vi "fill the pulse memory 4 memorys.vi"(10 "memory units":T1={"Memory In"="pulse on memory", "Memory In 2"="", "Memory In 3"="", "Memory In 6"="pulse on memory"}, 11 "FIFO In":refnum<k21>="fifo pulse from host") -> ()   [LabVIEW 2021]
uses:
  <vilib>/rvi/DataTransferAndStorage/Container/Common/niFpgaContainerExecOnDevCompGetState.vi
  <vilib>/rvi/Emulation/niFpgaEmulationIsFPGAContextNoSignature.vi
  <vilib>/rvi/Emulation/niFpgaSctlEmulationGetInTimedLoop.vi
  <vilib>/rvi/errors/niFpgaSetErrorForExecOnDevCompSimple.vi
  <vilib>/rvi/eio/common/nirviEmuReportErrorAndStop.vi
  <vilib>/rvi/DataTransferAndStorage/Container/Common/niFpgaContainerGetUniqueNameForEmu.vi
  <vilib>/rvi/FIFO/Fifo_Resource/nirvififoEmulationSetSize.vi
  <vilib>/rvi/FIFO/Fifo_Resource/nirviFifoEmulationQueueMgr.vi
  <instcachedir>/0/nirviFifoEmulationQueueMgr_E5CAEC123FF24DC58D834DCA3CDAA9B5.lvgen/nirviFifoEmulationQueueMgr_E5CAEC123FF24DC58D834DCA3CDAA9B5_008.vi
  <vilib>/rvi/FIFO/Fifo_Resource/nirvififoEmulationDetermineInputValidOut.vi
  <vilib>/rvi/FIFO/Fifo_Resource/nirvififoEmulationCreateLock.vi
  <vilib>/rvi/Emulation/niFpgaProcessEmulError.vi
  <vilib>/rvi/FIFO/Fifo_Resource/nirvififoEmulationObtainLock.vi
  <vilib>/rvi/FIFO/Fifo_Resource/nirvififoEmulationReleaseLock.vi
  <vilib>/rvi/occurrence/nirviWaitOnOccurrenceBase.vi
  <vilib>/rvi/errors/nirviReportUnexpectedCaseInternalError.vi
  <vilib>/rvi/errors/nirviReportUnexpectedCaseInternalError (U32).vi
  <vilib>/Utility/error.llb/Clear Errors.vi
  <vilib>/rvi/interface/RandomDataEmulation/niFpgaRandomDataHandleErrors.vi
  <vilib>/rvi/Memory/Memory_Emulation/niFpgaMemoryEmulationCacheClearOnFirstRun.vi
  <vilib>/rvi/Memory/Memory_Emulation/nirvimemoryEmulationManagerCache_MakeExclusive.vi
  <vilib>/rvi/Memory/Memory_Emulation/niFpgaMemoryEmulationValidateCache.vi
  <vilib>/rvi/Memory/Memory_Emulation/nirvimemoryEmulationManagerCache_InsertValue.vi
  <vilib>/rvi/Memory/Memory_Emulation/nirvimemoryEmulationManagerCache_ReleaseExclusive.vi
  <vilib>/rvi/Memory/Memory_Emulation/nirvimemoryEmulationManagerCache_GetValue.vi
  <vilib>/rvi/Memory/Memory_Emulation/nirvimemoryEmulationManagerCache_SetValue.vi
  <vilib>/rvi/Emulation/niFpgaSctlEmulationResourceMgr.vi
  <vilib>/rvi/DataTransferAndStorage/Container/XNode/niFpgaContainer.xnode
  <vilib>/rvi/FIFO/Fifo_Resource/niFpgaFifoEmulationRefIn.vi
  <vilib>/rvi/Memory/Memory_Emulation/niFpgaMemoryEmulationRefIn.vi
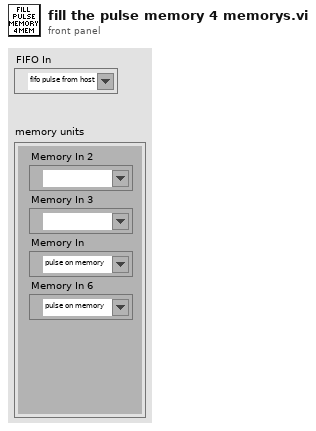
[diagram p1: front panel]
types:
  T1 = cluster{"Memory In":refnum<k21>, "Memory In 2":refnum<k21>, "Memory In 3":refnum<k21>, "Memory In 6":refnum<k21>}
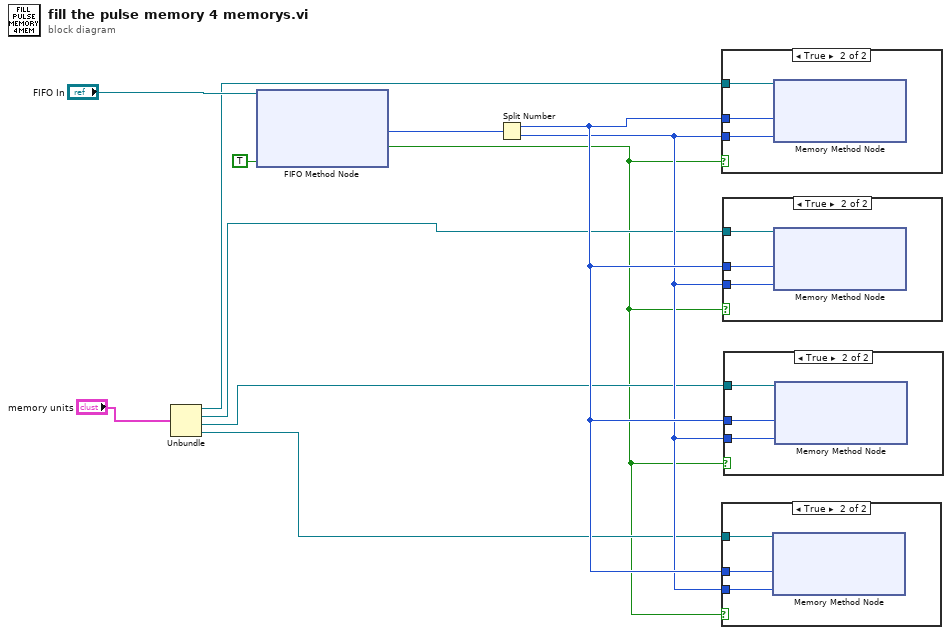
[diagram p0: block diagram]
diagram:
  n1 = Unbundle("memory units") -> ("Memory In"=w5:refnum<k21>, "Memory In 2"=w4:refnum<k21>, "Memory In 3"=w3:refnum<k21>, "Memory In 6"=w2:refnum<k21>)
  n2 = xnode ("FIFO Method Node")("Ready for Output"=TRUE, "FIFO In"="FIFO In") -> ("Element"=w11:u64, "Output Valid"=w1:bool)  [unwired: 1 out]
  n3 = Split Number(x=w11) -> (hi(x)=w8:u32, lo(x)=w7:u32)
  n4 = case shown="True" w1 {
    tunnel: w8 -> [_ w14]
    tunnel: w7 -> [_ w13]
    tunnel: w5 -> [_ w12]
    frame False {
    }
    frame True {
      n5 = xnode ("Memory Method Node")("Address"=w14, "Data"=w13, "Memory In"=w12) -> ()  [unwired: 1 out]
    }
  }
  n6 = case shown="True" w1 {
    tunnel: w8 -> [_ w17]
    tunnel: w7 -> [_ w16]
    tunnel: w2 -> [_ w15]
    frame False {
    }
    frame True {
      n7 = xnode ("Memory Method Node")("Address"=w17, "Data"=w16, "Memory In"=w15) -> ()  [unwired: 1 out]
    }
  }
  n8 = case shown="True" w1 {
    tunnel: w8 -> [_ w20]
    tunnel: w7 -> [_ w19]
    tunnel: w4 -> [_ w18]
    frame False {
    }
    frame True {
      n9 = xnode ("Memory Method Node")("Address"=w20, "Data"=w19, "Memory In"=w18) -> ()  [unwired: 1 out]
    }
  }
  n10 = case shown="True" w1 {
    tunnel: w8 -> [_ w23]
    tunnel: w7 -> [_ w22]
    tunnel: w3 -> [_ w21]
    frame False {
    }
    frame True {
      n11 = xnode ("Memory Method Node")("Address"=w23, "Data"=w22, "Memory In"=w21) -> ()  [unwired: 1 out]
    }
  }
